vi "dfd_Validate Filter Coef.vi"(8 "error in (no error)":errorcluster, 10 "coef source":enum16{"Original", "Current", "Quantized"}(ring)=enum."Current", 11 "filter in":T1={"mSRate_Fs"=1.0, "mSRate_Version"="1.0", "mSRate_Comments"="", "mSRate_OrgCoef"={"type"=enum."Undefined", "gain"=1.0, "coef a (k)"=[], "coef b (v)"=[]}, "mSRate_CurCoef"={"type"=enum."Undefined", "gain"=1.0, "coef a (k)"=[], "coef b (v)"=[]}, "mSRate_Quantized?"=FALSE, "mSRate_QCoef"={"type"=enum."Undefined", "gain"=1.0, "coef a (k)"=[], "coef b (v)"=[]}, "mSRate_QSettings"=[], "mSRate_Order"=0, "mSRate_Scaling"={"mSRate_ScaleByPowerOf2?"=FALSE, "mSRate_ScaleType"=enum."No Norm"}} {"mSRate_QSettings"."source" items=["Coef a/k"=0, "Coef b/v"=7, "Input"=1, "Output"=2, "Multiplicand"=3, "Product"=4, "Sum"=5, "Delay"=6, "Gain"=8]}) -> (0 "error out":errorcluster, 2 "is Valid?":bool, 3 "filter out":T1={"mSRate_Fs"=1.0, "mSRate_Version"="1.0", "mSRate_Comments"="", "mSRate_OrgCoef"={"type"=enum."Undefined", "gain"=1.0, "coef a (k)"=[], "coef b (v)"=[]}, "mSRate_CurCoef"={"type"=enum."Undefined", "gain"=1.0, "coef a (k)"=[], "coef b (v)"=[]}, "mSRate_Quantized?"=FALSE, "mSRate_QCoef"={"type"=enum."Undefined", "gain"=1.0, "coef a (k)"=[], "coef b (v)"=[]}, "mSRate_QSettings"=[], "mSRate_Order"=0, "mSRate_Scaling"={"mSRate_ScaleByPowerOf2?"=FALSE, "mSRate_ScaleType"=enum."No Norm"}} {"mSRate_QSettings"."source" items=["Coef a/k"=0, "Coef b/v"=7, "Input"=1, "Output"=2, "Multiplicand"=3, "Product"=4, "Sum"=5, "Delay"=6, "Gain"=8]})   [LabVIEW 2017, in "NI_DigFilterLicensed.lvlib"]
uses:
  <vilib>/addons/Digital Filter Design/NI_DigFilterLicensed.lvlib
  <vilib>/addons/Digital Filter Design/_Objects.llb/DFD Filter Obj.ctl
  <vilib>/addons/Digital Filter Design/_Objects.llb/DFD Filter Coef.ctl
  <vilib>/addons/Digital Filter Design/_Objects.llb/DFD Filter Structure Type Selector.ctl
  <vilib>/addons/Digital Filter Design/_Objects.llb/dfd_Internal Quantization Settings.ctl
  <vilib>/addons/Digital Filter Design/_Objects.llb/dfd_Internal Quantization Srcs.ctl
  <vilib>/addons/Digital Filter Design/_Objects.llb/DFD Coef Norm Type.ctl
  <vilib>/addons/Digital Filter Design/_Misc.llb/dfd_Error Handlers (Multiple).vi
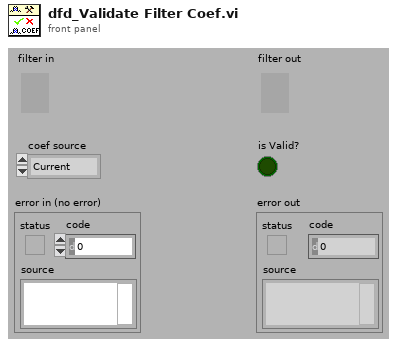
[diagram p1: front panel]
types:
  T1 = typedef "NI_DigFilterLicensed.lvlib/DFD Filter Obj.ctl" = cluster{"mSRate_Fs":dbl, "mSRate_Version":string, "mSRate_Comments":string, "mSRate_OrgCoef":T2, "mSRate_CurCoef":T2, "mSRate_Quantized?":bool, "mSRate_QCoef":T2, "mSRate_QSettings":T4[], "mSRate_Order":i32, "mSRate_Scaling":cluster{"mSRate_ScaleByPowerOf2?":bool, "mSRate_ScaleType":T6}}
  T2 = typedef "NI_DigFilterLicensed.lvlib/DFD Filter Coef.ctl" = cluster{"type":T3, "gain":dbl, "coef a (k)":dbl[], "coef b (v)":dbl[]}
  T3 = typedef "NI_DigFilterLicensed.lvlib/DFD Filter Structure Type Selector.ctl" = enum16{"Undefined", "FIR Direct Form", "FIR Direct Form Transposed", "FIR Symmetric", "FIR Antisymmetric", "IIR Direct Form I", "IIR Direct Form I Transposed", "IIR Direct Form II", "IIR Direct Form II Transposed", "IIR Cascaded Second Order Sections Form I", "IIR Cascaded Second Order Sections Form I Transposed", "IIR Cascaded Second Order Sections Form II", "IIR Cascaded Second Order Sections Form II Transposed", "Lattice Allpass (basic sections)", "Lattice Allpass (one multiplier sections)", "Lattice Allpass (normalized sections)", "Lattice AR (basic sections)", "Lattice AR (one multiplier sections)", "Lattice AR (normalized sections)", "Lattice MA (minimum phase)", "Lattice MA (maximum phase)", "Lattice ARMA (basic sections)", "Lattice ARMA (one multiplier sections)", "Lattice ARMA (normalized sections)"}
  T4 = typedef "NI_DigFilterLicensed.lvlib/dfd_Internal Quantization Settings.ctl" = cluster{"source":T5, "wl":i16, "iwl":i16, "overflow mode":enum16{"Saturation", "Wrap"}, "rounding mode":enum16{"Nearest", "Truncation"}, "signed?":bool}
  T5 = typedef "NI_DigFilterLicensed.lvlib/dfd_Internal Quantization Srcs.ctl" = u16
  T6 = typedef "NI_DigFilterLicensed.lvlib/DFD Coef Norm Type.ctl" = enum16{"No Norm", "Time Domain 1-Norm", "Time Domain 2-Norm", "Time Domain Inf-Norm"}
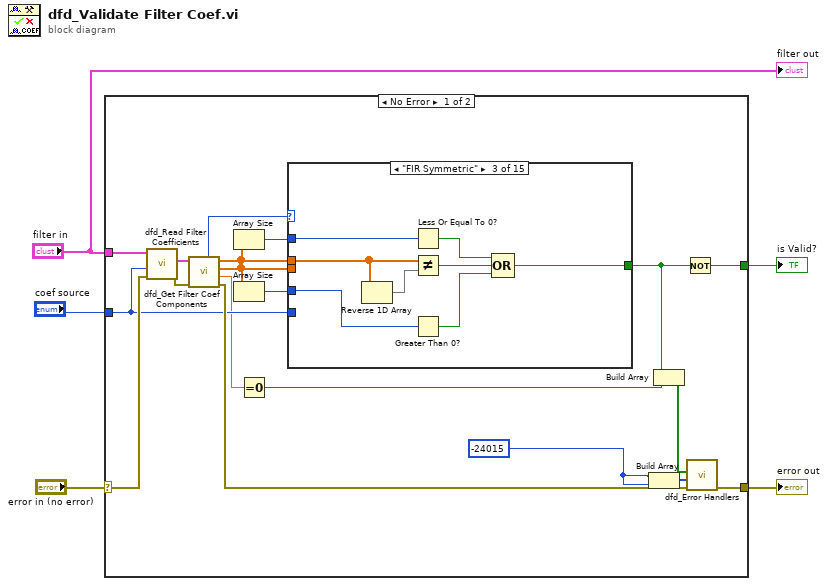
[diagram p0: block diagram]
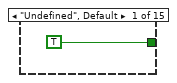
[diagram p2: hidden frame]
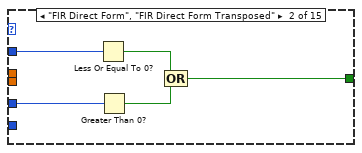
[diagram p3: hidden frame]
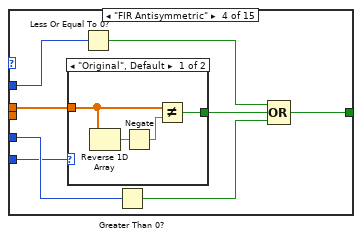
[diagram p4: hidden frame]
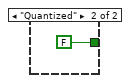
[diagram p5: hidden frame]
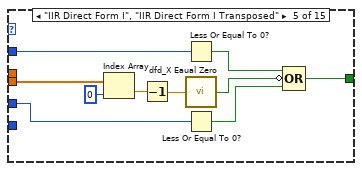
[diagram p6: hidden frame]
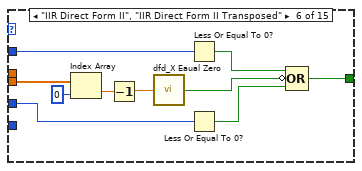
[diagram p7: hidden frame]
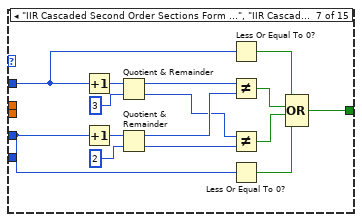
[diagram p8: hidden frame]
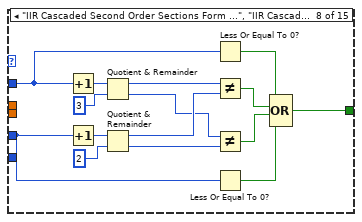
[diagram p9: hidden frame]
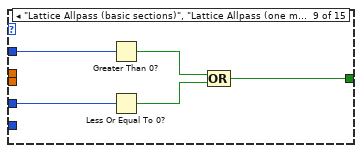
[diagram p10: hidden frame]
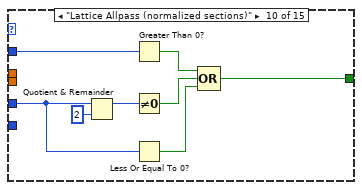
[diagram p11: hidden frame]
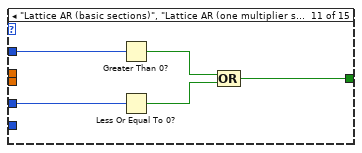
[diagram p12: hidden frame]
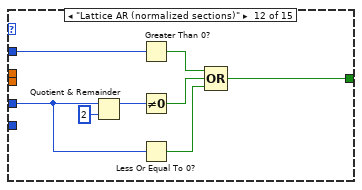
[diagram p13: hidden frame]
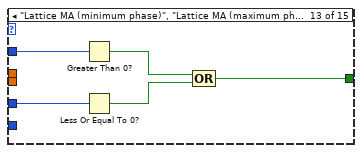
[diagram p14: hidden frame]
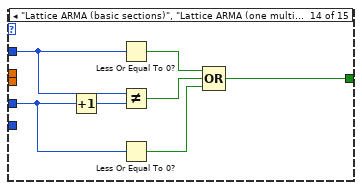
[diagram p15: hidden frame]
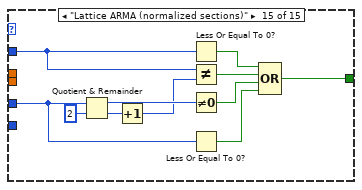
[diagram p16: hidden frame]
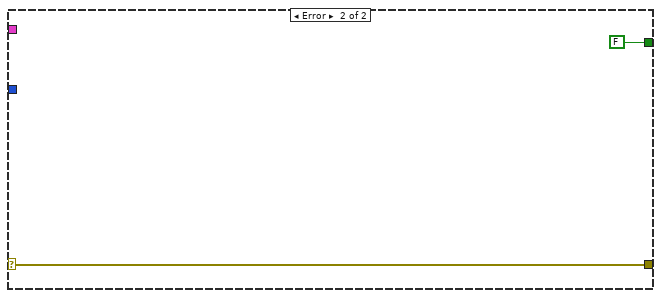
[diagram p17: hidden frame]
diagram:
  n1 = case shown="No Error" "error in (no error)" {
    selector: "error in (no error)" -> [w20 w152]
    tunnel: [w14 w152] -> w5
    tunnel: "filter in" -> [w24 _]
    tunnel: "coef source" -> [w13 _]
    tunnel: [w11 FALSE] -> w1
    frame No Error {
      w7 = -24015 ("ERR_INVALID_FILTER_OBJ")
      n2 = call <vilib>:"dfd_Read Filter Coefficients.vi"("error in (no error)"=w20, "coef source"=w13, "filter in"=w24) -> ("error out"=w22:errorcluster, "filter coef"=w23:T2)  [unwired: 7 out]
      n3 = call <vilib>:"dfd_Get Filter Coef Components.vi"("error in (no error)"=w22, "filter coef"=w23) -> ("error out"=w15:errorcluster, "gain"=w9:dbl, "coef a (k)"=w18:dbl[], "coef b (v)"=w19:dbl[], "type"=w21:T3)  [unwired: 5 out]
      n4 = Array Size(array=w19) -> (size(s)=w17:i32)
      n5 = Array Size(array=w18) -> (size(s)=w16:i32)
      n6 = Equal To 0?(x=w9) -> (x = 0?=w8:bool)
      n7 = case shown="\"FIR Symmetric\"" w21 {
        tunnel: w19 -> [_ _ w37 w43 _ _ _ _ _ _ _ _ _ _ _]
        tunnel: w18 -> [_ _ _ _ w58 w64 _ _ _ _ _ _ _ _ _]
        tunnel: w17 -> [_ w30 w36 w41 w57 w66 w80 w89 w105 w109 w117 w122 w132 w136 w146]
        tunnel: w16 -> [_ w29 w35 w40 w56 w65 w79 w88 w106 w110 w116 w121 w131 w138 w145]
        tunnel: [TRUE w26 w31 w42 w55 w63 w72 w87 w104 w107 w115 w120 w128 w133 w140] -> w12
        tunnel: w13 -> [_ _ _ w39 _ _ _ _ _ _ _ _ _ _ _]
        frame "Undefined", Default {
        }
        frame "FIR Direct Form", "FIR Direct Form Transposed" {
          n8 = Less Or Equal To 0?(x=w30) -> (x <= 0?=w28:bool)
          n9 = Greater Than 0?(x=w29) -> (x > 0?=w27:bool)
          n10 = Compound Arithmetic op=OR(w28, w27) -> (w26:bool)
        }
        frame "FIR Symmetric" {
          n11 = Reverse 1D Array(array=w37) -> (reversed array=w38:dbl[])
          n12 = Less Or Equal To 0?(x=w36) -> (x <= 0?=w34:bool)
          n13 = Not Equal?(x=w37, y=w38) -> (x != y?=w33:bool)
          n14 = Greater Than 0?(x=w35) -> (x > 0?=w32:bool)
          n15 = Compound Arithmetic op=OR(w34, w33, w32) -> (w31:bool)
        }
        frame "FIR Antisymmetric" {
          n16 = case shown="\"Original\", Default" w39 {
            tunnel: [w49 FALSE] -> w45
            tunnel: w43 -> [w48 _]
            frame "Original", Default {
              n17 = Reverse 1D Array(array=w48) -> (reversed array=w50:dbl[])
              n18 = Negate(x=w50) -> (-x=w47:dbl[])
              n19 = Not Equal?(x=w48, y=w47) -> (x != y?=w49:bool)
            }
            frame "Quantized" {
            }
          }
          n20 = Less Or Equal To 0?(x=w41) -> (x <= 0?=w46:bool)
          n21 = Greater Than 0?(x=w40) -> (x > 0?=w44:bool)
          n22 = Compound Arithmetic op=OR(w46, w45, w44) -> (w42:bool)
        }
        frame "IIR Direct Form I", "IIR Direct Form I Transposed" {
          n23 = Index Array(array=w58, index=0) -> (element=w60:dbl)
          n24 = Decrement(x=w60) -> (x-1=w52:dbl)
          n25 = Less Or Equal To 0?(x=w57) -> (x <= 0?=w54:bool)
          n26 = call <vilib>:"dfd_X Eaual Zero.vi"("x"=w52) -> ("equal?"=w59:bool)  [unwired: 1 in]
          n27 = Less Or Equal To 0?(x=w56) -> (x <= 0?=w53:bool)
          n28 = Compound Arithmetic op=OR(w54, invert w59, w53) -> (w55:bool)
        }
        frame "IIR Direct Form II", "IIR Direct Form II Transposed" {
          n29 = Index Array(array=w64, index=0) -> (element=w70:dbl)
          n30 = Decrement(x=w70) -> (x-1=w62:dbl)
          n31 = call <vilib>:"dfd_X Eaual Zero.vi"("x"=w62) -> ("equal?"=w69:bool)  [unwired: 1 in]
          n32 = Less Or Equal To 0?(x=w66) -> (x <= 0?=w68:bool)
          n33 = Less Or Equal To 0?(x=w65) -> (x <= 0?=w67:bool)
          n34 = Compound Arithmetic op=OR(w68, invert w69, w67) -> (w63:bool)
        }
        frame "IIR Cascaded Second Order Sections Form I", "IIR Cascaded Second Order Sections Form I Transposed" {
          n35 = Increment(x=w80) -> (x+1=w83:i32)
          n36 = Increment(x=w79) -> (x+1=w84:i32)
          n37 = Quotient & Remainder(x=w83, y=3) -> (x-y*floor(x/y)=w78:i32, floor(x/y)=w75:i32)
          n38 = Quotient & Remainder(x=w84, y=2) -> (x-y*floor(x/y)=w77:i32, floor(x/y)=w76:i32)
          n39 = Less Or Equal To 0?(x=w80) -> (x <= 0?=w82:bool)
          n40 = Not Equal?(x=w78, y=w77) -> (x != y?=w73:bool)
          n41 = Not Equal?(x=w75, y=w76) -> (x != y?=w74:bool)
          n42 = Less Or Equal To 0?(x=w79) -> (x <= 0?=w81:bool)
          n43 = Compound Arithmetic op=OR(w82, w73, w74, w81) -> (w72:bool)
        }
        frame "IIR Cascaded Second Order Sections Form II", "IIR Cascaded Second Order Sections Form II Transposed" {
          n44 = Increment(x=w89) -> (x+1=w98:i32)
          n45 = Increment(x=w88) -> (x+1=w99:i32)
          n46 = Quotient & Remainder(x=w98, y=3) -> (x-y*floor(x/y)=w95:i32, floor(x/y)=w92:i32)
          n47 = Quotient & Remainder(x=w99, y=2) -> (x-y*floor(x/y)=w94:i32, floor(x/y)=w93:i32)
          n48 = Less Or Equal To 0?(x=w89) -> (x <= 0?=w97:bool)
          n49 = Not Equal?(x=w95, y=w94) -> (x != y?=w90:bool)
          n50 = Not Equal?(x=w92, y=w93) -> (x != y?=w91:bool)
          n51 = Less Or Equal To 0?(x=w88) -> (x <= 0?=w96:bool)
          n52 = Compound Arithmetic op=OR(w97, w90, w91, w96) -> (w87:bool)
        }
        frame "Lattice Allpass (basic sections)", "Lattice Allpass (one multiplier sections)" {
          n53 = Greater Than 0?(x=w105) -> (x > 0?=w103:bool)
          n54 = Less Or Equal To 0?(x=w106) -> (x <= 0?=w102:bool)
          n55 = Compound Arithmetic op=OR(w103, w102) -> (w104:bool)
        }
        frame "Lattice Allpass (normalized sections)" {
          n56 = Quotient & Remainder(x=w110, y=2) -> (x-y*floor(x/y)=w113:i32)  [unwired: 1 out]
          n57 = Greater Than 0?(x=w109) -> (x > 0?=w112:bool)
          n58 = Not Equal To 0?(x=w113) -> (x != 0?=w111:bool)
          n59 = Less Or Equal To 0?(x=w110) -> (x <= 0?=w108:bool)
          n60 = Compound Arithmetic op=OR(w112, w111, w108) -> (w107:bool)
        }
        frame "Lattice AR (basic sections)", "Lattice AR (one multiplier sections)" {
          n61 = Greater Than 0?(x=w117) -> (x > 0?=w119:bool)
          n62 = Less Or Equal To 0?(x=w116) -> (x <= 0?=w118:bool)
          n63 = Compound Arithmetic op=OR(w119, w118) -> (w115:bool)
        }
        frame "Lattice AR (normalized sections)" {
          n64 = Quotient & Remainder(x=w121, y=2) -> (x-y*floor(x/y)=w126:i32)  [unwired: 1 out]
          n65 = Greater Than 0?(x=w122) -> (x > 0?=w125:bool)
          n66 = Not Equal To 0?(x=w126) -> (x != 0?=w124:bool)
          n67 = Less Or Equal To 0?(x=w121) -> (x <= 0?=w123:bool)
          n68 = Compound Arithmetic op=OR(w125, w124, w123) -> (w120:bool)
        }
        frame "Lattice MA (minimum phase)", "Lattice MA (maximum phase)" {
          n69 = Greater Than 0?(x=w132) -> (x > 0?=w130:bool)
          n70 = Less Or Equal To 0?(x=w131) -> (x <= 0?=w129:bool)
          n71 = Compound Arithmetic op=OR(w130, w129) -> (w128:bool)
        }
        frame "Lattice ARMA (basic sections)", "Lattice ARMA (one multiplier sections)" {
          n72 = Increment(x=w138) -> (x+1=w137:i32)
          n73 = Less Or Equal To 0?(x=w136) -> (x <= 0?=w135:bool)
          n74 = Not Equal?(x=w136, y=w137) -> (x != y?=w139:bool)
          n75 = Less Or Equal To 0?(x=w138) -> (x <= 0?=w134:bool)
          n76 = Compound Arithmetic op=OR(w135, w139, w134) -> (w133:bool)
        }
        frame "Lattice ARMA (normalized sections)" {
          n77 = Quotient & Remainder(x=w145, y=2) -> (x-y*floor(x/y)=w149:i32, floor(x/y)=w148:i32)
          n78 = Increment(x=w148) -> (x+1=w147:i32)
          n79 = Less Or Equal To 0?(x=w146) -> (x <= 0?=w144:bool)
          n80 = Not Equal?(x=w146, y=w147) -> (x != y?=w143:bool)
          n81 = Not Equal To 0?(x=w149) -> (x != 0?=w142:bool)
          n82 = Less Or Equal To 0?(x=w145) -> (x <= 0?=w141:bool)
          n83 = Compound Arithmetic op=OR(w144, w143, w142, w141) -> (w140:bool)
        }
      }
      n84 = Build Array(w7, w7) -> (w6:i32[])
      n85 = Build Array(w12, w8) -> (w10:bool[])
      n86 = Not(x=w12) -> (.not. x?=w11:bool)
      n87 = call-poly <vilib>:"dfd_Error Handlers.vi"("error in (no error)"=w15, "error sources"=w6, "condition failed?"=w10) -> ("error out"=w14:errorcluster)  [unwired: 8 out]
    }
    frame Error {
    }
  }
  "error out" <- w5
  "is Valid?" <- w1
  "filter out" <- "filter in"
